vi "ConvertConfigCluster.vi"(10 "Original Board Control In":T4 {"Port1ConfigIn" items=["FDX_SINGLE", "FDX_REDUNDANT"]; "Port2ConfigIn" items=["FDX_SINGLE", "FDX_REDUNDANT"]; "Port3ConfigIn" items=["FDX_SINGLE", "FDX_REDUNDANT"]; "Port4ConfigIn" items=["FDX_SINGLE", "FDX_REDUNDANT"]; "Port1SpeedIn" items=["FDX_100MBIT", "FDX_10MBIT", "FDX_AUTO_100MBIT", "FDX_AUTO_10MBIT", "FDX_1000MBIT"]; "Port2SpeedIn" items=["FDX_100MBIT", "FDX_10MBIT", "FDX_AUTO_100MBIT", "FDX_AUTO_10MBIT", "FDX_1000MBIT"]; "Port3SpeedIn" items=["FDX_100MBIT", "FDX_10MBIT", "FDX_AUTO_100MBIT", "FDX_AUTO_10MBIT", "FDX_1000MBIT"]; "Port4SpeedIn" items=["FDX_100MBIT", "FDX_10MBIT", "FDX_AUTO_100MBIT", "FDX_AUTO_10MBIT", "FDX_1000MBIT"]; "Expert1Mode" items=["FDX_EXPERT_MODE", "FDX_DISA_GHOST"]; "Expert2Mode" items=["FDX_EXPERT_MODE", "FDX_DISA_GHOST"]; "Expert3Mode" items=["FDX_EXPERT_MODE", "FDX_DISA_GHOST"]; "Expert4Mode" items=["FDX_EXPERT_MODE", "FDX_DISA_GHOST"]}, 11 "Board Control Output":T6 {"PortConfig" items=["FDX_SINGLE", "FDX_REDUNDANT"]; "PortSpeed" items=["FDX_100MBIT", "FDX_10MBIT", "FDX_AUTO_100MBIT", "FDX_AUTO_10MBIT", "FDX_1000MBIT"]; "PortGoodLink" items=["FDX_NO_LINK", "FDX_GOOD_LINK"]; "ExpertMode" items=["FDX_EXPERT_MODE", "FDX_DISA_GHOST"]}) -> (3 "Adjusted Board Control Input":T4 {"Port1ConfigIn" items=["FDX_SINGLE", "FDX_REDUNDANT"]; "Port2ConfigIn" items=["FDX_SINGLE", "FDX_REDUNDANT"]; "Port3ConfigIn" items=["FDX_SINGLE", "FDX_REDUNDANT"]; "Port4ConfigIn" items=["FDX_SINGLE", "FDX_REDUNDANT"]; "Port1SpeedIn" items=["FDX_100MBIT", "FDX_10MBIT", "FDX_AUTO_100MBIT", "FDX_AUTO_10MBIT", "FDX_1000MBIT"]; "Port2SpeedIn" items=["FDX_100MBIT", "FDX_10MBIT", "FDX_AUTO_100MBIT", "FDX_AUTO_10MBIT", "FDX_1000MBIT"]; "Port3SpeedIn" items=["FDX_100MBIT", "FDX_10MBIT", "FDX_AUTO_100MBIT", "FDX_AUTO_10MBIT", "FDX_1000MBIT"]; "Port4SpeedIn" items=["FDX_100MBIT", "FDX_10MBIT", "FDX_AUTO_100MBIT", "FDX_AUTO_10MBIT", "FDX_1000MBIT"]; "Expert1Mode" items=["FDX_EXPERT_MODE", "FDX_DISA_GHOST"]; "Expert2Mode" items=["FDX_EXPERT_MODE", "FDX_DISA_GHOST"]; "Expert3Mode" items=["FDX_EXPERT_MODE", "FDX_DISA_GHOST"]; "Expert4Mode" items=["FDX_EXPERT_MODE", "FDX_DISA_GHOST"]})   [LabVIEW 2020, in "AIM664LV.lvlib"]
uses:
  _controls/port_configuration.ctl
  _controls/port_speed.ctl
  _controls/expert_mode.ctl
  _controls/port_condition.ctl
  AIM664LV.lvlib
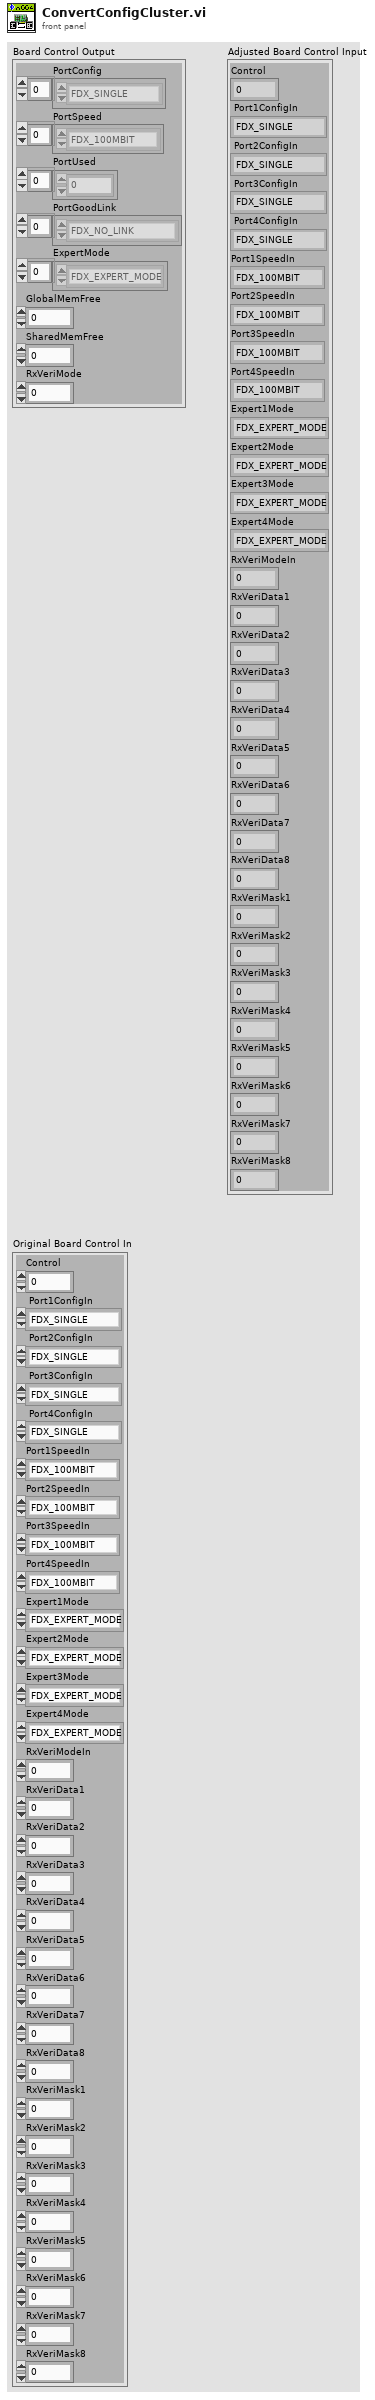
[diagram p1: front panel]
types:
  T1 = typedef "AIM664LV.lvlib/port_configuration.ctl" = u32
  T2 = typedef "AIM664LV.lvlib/port_speed.ctl" = u32
  T3 = typedef "AIM664LV.lvlib/expert_mode.ctl" = u32
  T4 = cluster{"Control":u32, "Port1ConfigIn":T1, "Port2ConfigIn":T1, "Port3ConfigIn":T1, "Port4ConfigIn":T1, "Port1SpeedIn":T2, "Port2SpeedIn":T2, "Port3SpeedIn":T2, "Port4SpeedIn":T2, "Expert1Mode":T3, "Expert2Mode":T3, "Expert3Mode":T3, "Expert4Mode":T3, "RxVeriModeIn":u32, "RxVeriData1":u32, "RxVeriData2":u32, "RxVeriData3":u32, "RxVeriData4":u32, "RxVeriData5":u32, "RxVeriData6":u32, "RxVeriData7":u32, "RxVeriData8":u32, "RxVeriMask1":u32, "RxVeriMask2":u32, "RxVeriMask3":u32, "RxVeriMask4":u32, "RxVeriMask5":u32, "RxVeriMask6":u32, "RxVeriMask7":u32, "RxVeriMask8":u32}
  T5 = typedef "AIM664LV.lvlib/port_condition.ctl" = u32
  T6 = cluster{"PortConfig":T1[], "PortSpeed":T2[], "PortUsed":u32[], "PortGoodLink":T5[], "ExpertMode":T3[], "GlobalMemFree":u32, "SharedMemFree":u32, "RxVeriMode":u32}
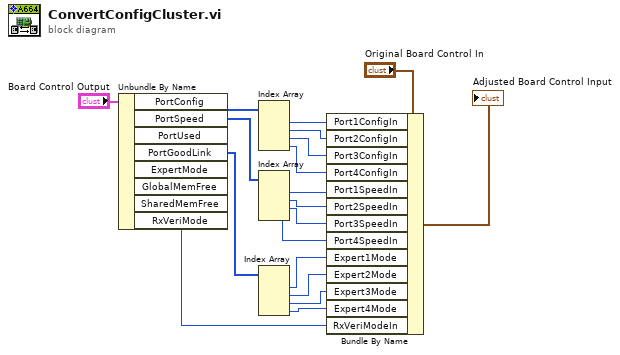
[diagram p0: block diagram]
diagram:
  n1 = Unbundle By Name("Board Control Output") -> ("PortConfig"=w16:T1[], "PortSpeed"=w11:T2[], "PortGoodLink"=w6:T5[], "RxVeriMode"=w1:u32)  [unwired: 4 out]
  n2 = Index Array(array=w16) -> (element #1=w15:T1, element #2=w14:T1, element #3=w13:T1, element #4=w12:T1)  [unwired: 4 in]
  n3 = Index Array(array=w11) -> (element #1=w10:T2, element #2=w9:T2, element #3=w8:T2, element #4=w7:T2)  [unwired: 4 in]
  n4 = Index Array(array=w6) -> (element #1=w5:T5, element #2=w4:T5, element #3=w3:T5, element #4=w2:T5)  [unwired: 4 in]
  n5 = Bundle By Name(cluster="Original Board Control In", "Port1ConfigIn"=w15, "Port2ConfigIn"=w14, "Port3ConfigIn"=w13, "Port4ConfigIn"=w12, "Port1SpeedIn"=w10, "Port2SpeedIn"=w9, "Port3SpeedIn"=w8, "Port4SpeedIn"=w7, "Expert1Mode"=w5, "Expert2Mode"=w4, "Expert3Mode"=w3, "Expert4Mode"=w2, "RxVeriModeIn"=w1) -> (→"Adjusted Board Control Input":T4)
